vi "系统设置.vi"() -> ()   [LabVIEW 2016]
uses:
  <vilib>/Utility/miscctls.llb/LVPointTypeDef.ctl
  <vilib>/Utility/config.llb/Read Key (U32).vi
  <vilib>/Utility/config.llb/Write Key (I32).vi
  PLC/PLC.lvlib
  <vilib>/ptbypt/NI_PtbyPt.lvlib
  <vilib>/Utility/config.llb/NI_LVConfig.lvlib
panel:
  in  "采水模式":enum16{"使用采水泵", "不使用采水泵"}(ring)
  in  "运行模式":enum16{"维护模式", "常规模式", "应急模式", "质控模式"}(ring)
  in  "运行间隔":i16=4 min=1 max=24
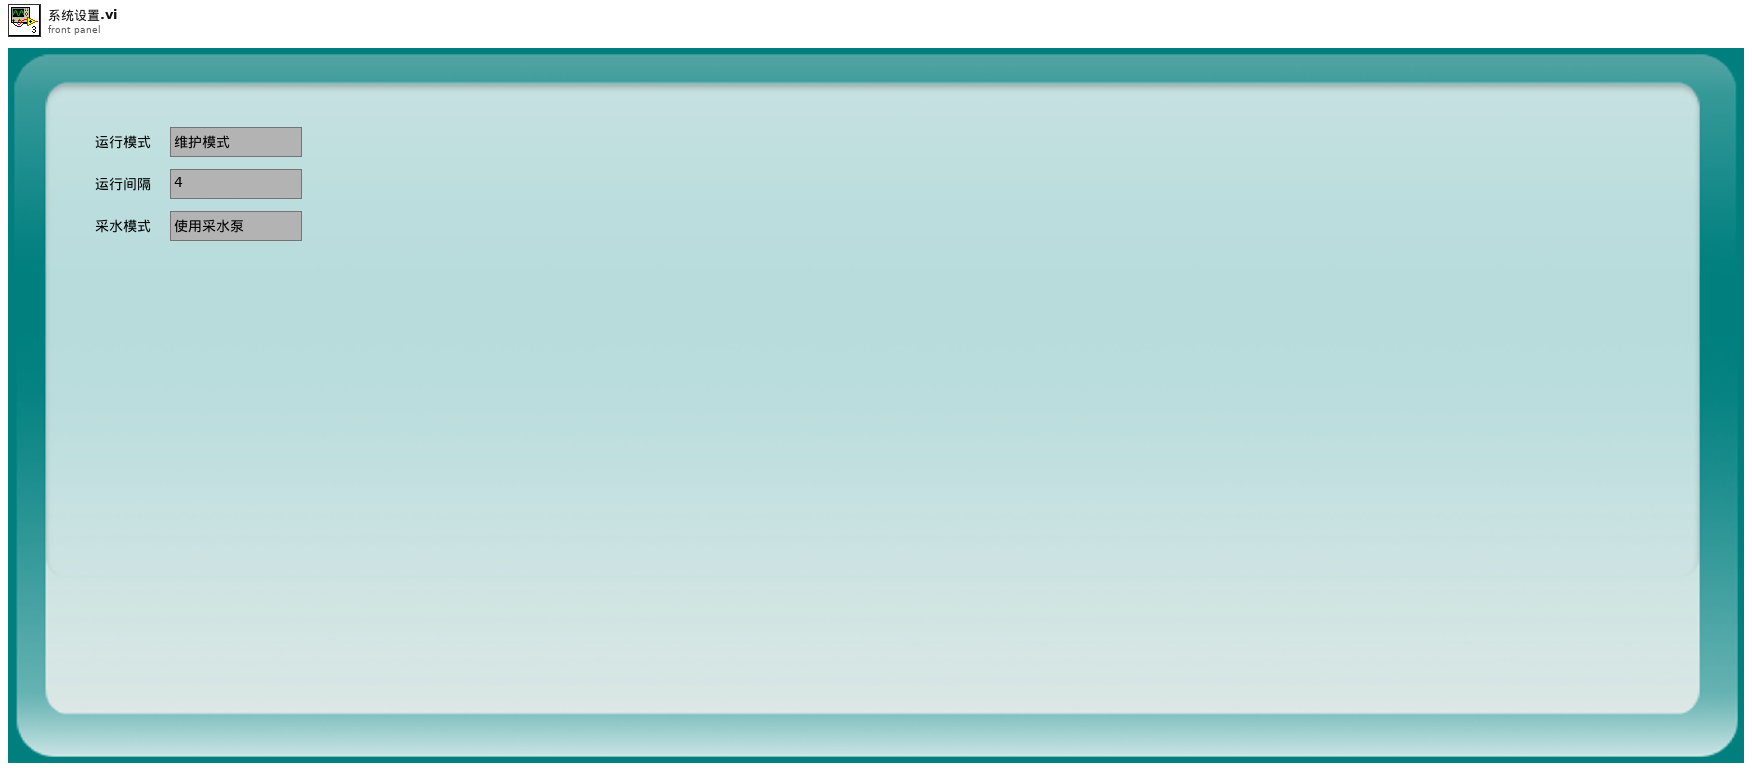
[diagram p1: front panel]
types:
  T1 = typedef "LVPointTypeDef.ctl" = cluster{"Horizontal":i16, "Vertical":i16}
  T2 = typedef "NI_LVConfig.lvlib/Config Data RefNum.ctl" = refnum<k1>
  T3 = enum16{"水样测量", "标样核查", "零点核查", "加标回收", "平行样", "校零", "校标"}
  T4 = cluster{"是否启用仪器":bool, "CODMn":cluster{"启动测量模式":cluster{"测量模式":enum16{"水样测量", "标样核查", "零点核查", "加标回收", "平行样", "校零", "校标"}}, "确定按钮":bool}, "CODCr":cluster{"启动测量模式":cluster{"测量模式":enum16{"水样测量", "标样核查", "零点核查", "加标回收", "平行样", "校零", "校标"}}}, "采水模式":enum16{"使用采水泵", "不使用采水泵"}}
  T5 = typedef "LVDateTimeRec.ctl" = cluster{"秒数的小数部分":dbl, "秒":i32, "分":i32, "时":i32, "日":i32, "月":i32, "年":i32, "天数（周）":i32, "天数（年）":i32, "DST":i32}
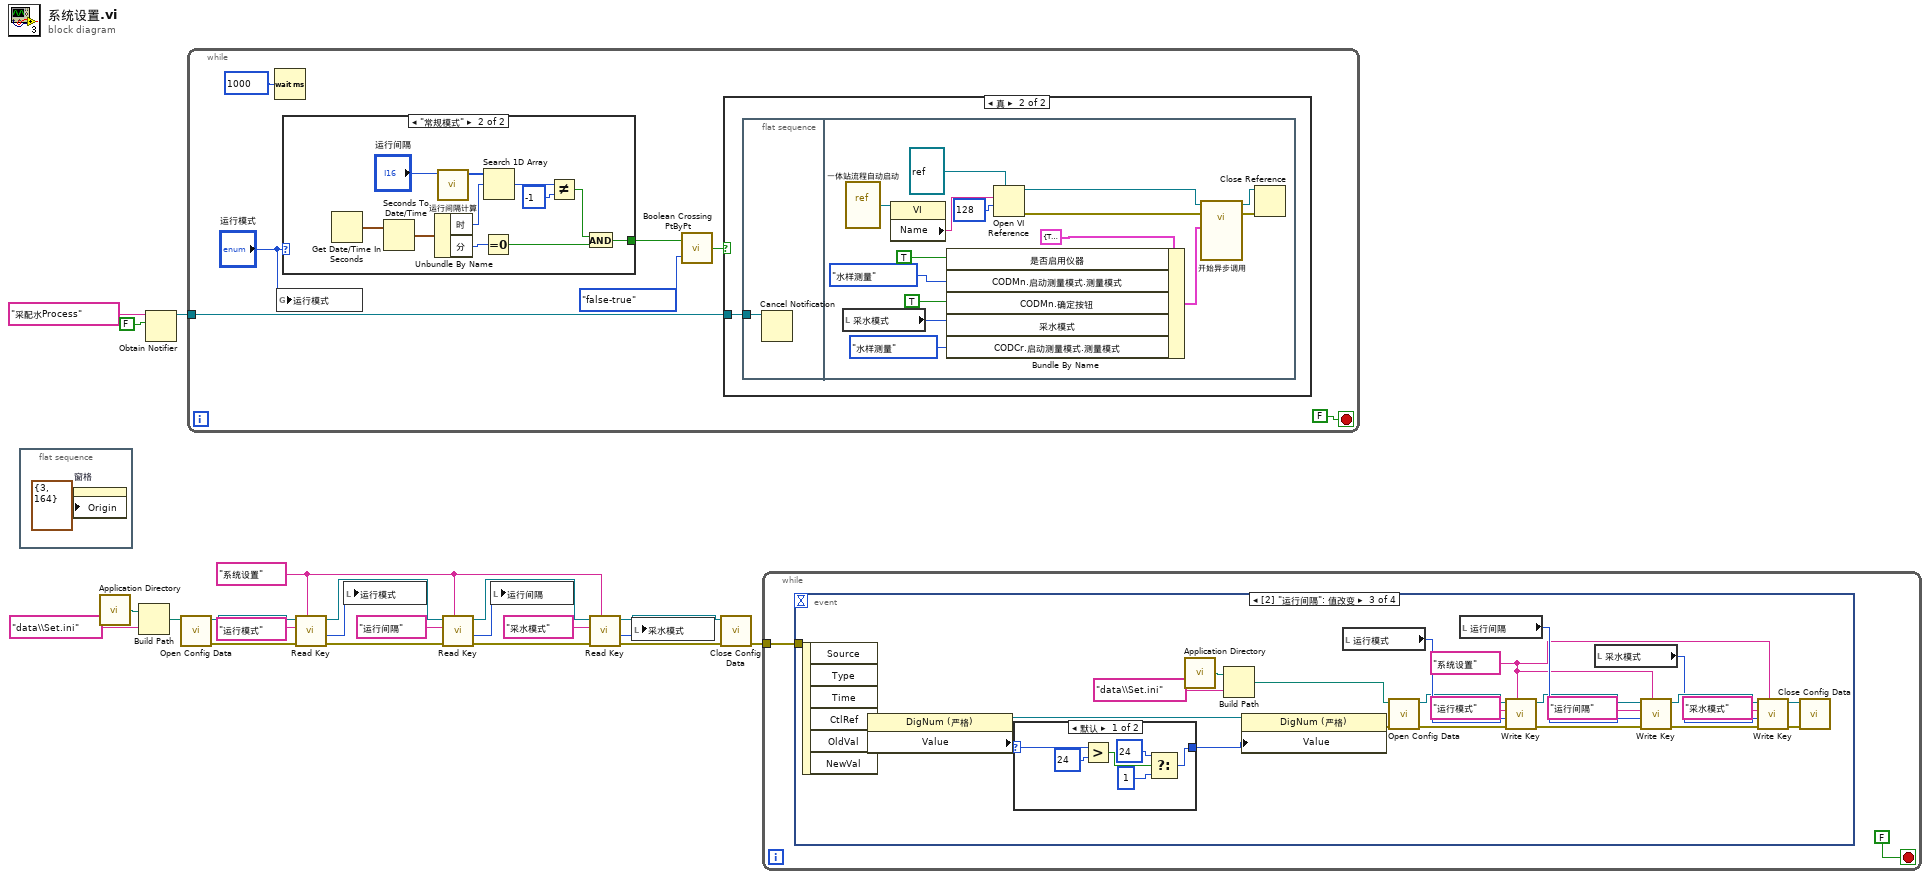
[diagram p0: block diagram]
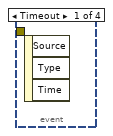
[diagram p4: hidden frame]
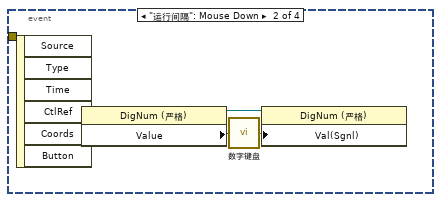
[diagram p5: hidden frame]
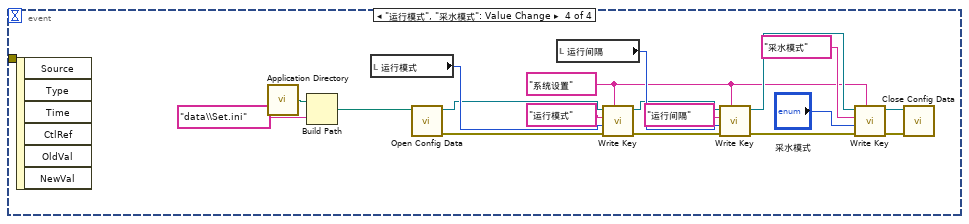
[diagram p7: hidden frame]
diagram:
  w3 = "系统设置" ("section")
  n1 = flat-sequence {
    frame #0 {
      n2 = property on="窗格" class="Pane"("Origin"=T1 {"Horizontal"=3, "Vertical"=164} ("原点")) -> ()  [unwired: 2 in, 2 out]
    }
  }
  n3 = call <vilib>:"Application Directory.vi"() -> ("Application Directory"=w17:path)
  n4 = Build Path(base path=w17, name or relative path="data\\Set.ini" ("名称或相对路径")) -> (appended path=w15:path)
  n5 = Obtain Notifier(name (unnamed)="采配水Process" ("名称（未命名）"), notification data type=FALSE) -> (notifier out=w20:refnum<notifier>)  [unwired: 2 in, 2 out]
  n6 = call <vilib>:"Open Config Data.vi"("configuration file path"=w15) -> ("error out"=w18:errorcluster, "refnum"=w19:T2)  [unwired: 8 in, 1 out]
  n7 = while {
    tunnel: w20 -> [w28]
    stop <- FALSE stop-if-true
    n8 = Wait (ms)(milliseconds to wait=u32 1000 ("等待时间（毫秒）")) -> ()  [unwired: 1 out]
    n9 = global write "系统变量.vi" "运行模式"("运行模式") -> ()
    n10 = case shown="\"常规模式\"" "运行模式" {
      tunnel: [_ w48] -> w27
      frame "维护模式", Default {
      }
      frame "常规模式" {
        n11 = Get Date/Time In Seconds() -> (seconds since 1Jan1904=w57:timestamp)
        n12 = Seconds To Date/Time(time stamp (now)=w57) -> (date time rec=w56:T5)  [unwired: 1 in]
        n13 = Unbundle By Name(w56) -> ("时"=w53:i32, "分"=w55:i32)
        n14 = call "运行间隔计算.vi"("运行周期"="运行间隔") -> ("数组"=w54:i32[])  [unwired: 10 in]
        n15 = Equal To 0?(x=w55) -> (x = 0?=w49:bool)
        n16 = Search 1D Array(1D array=w54, element=w53) -> (index of element=w52:i32)  [unwired: 1 in]
        n17 = Not Equal?(x=w52, y=-1) -> (x != y?=w50:bool)
        n18 = And(x=w50, y=w49) -> (x .and. y?=w48:bool)
      }
    }
    n19 = call <vilib>:"Boolean Crossing PtByPt.vi"("direction"=enum16{"either", "false-true", "true-false"}."false-true", "input"=w27) -> ("crossing"=w25:bool)  [unwired: 1 in]
    n20 = case shown="真" w25 {
      tunnel: w28 -> [_ w31]
      frame False {
      }
      frame True {
        n21 = flat-sequence {
          tunnel: w31 -> [w32]
          frame #0 {
            n22 = Cancel Notification(0:w32) -> ()  [unwired: 1 in, 3 out]
          }
          frame #1 {
            n23 = local read "采水模式"() -> (w36:enum16{"使用采水泵", "不使用采水泵"})
            n24 = vi-ref "一体站流程自动启动.vi"() -> (w47:refnum<vi>)
            n25 = property class="VI"(reference=w47) -> ("Name"=w46:string)  [unwired: 1 in, 2 out]
            n26 = Bundle By Name(cluster=T4 {"是否启用仪器"=TRUE, "CODMn"={"启动测量模式"={"测量模式"=enum."水样测量"}, "确定按钮"=TRUE}, "CODCr"={"启动测量模式"={"测量模式"=enum."水样测量"}}, "采水模式"=enum."使用采水泵"} ("参数"), "是否启用仪器"=TRUE, "CODMn.启动测量模式.测量模式"=T3."水样测量", "CODMn.确定按钮"=TRUE, "采水模式"=w36, "CODCr.启动测量模式.测量模式"=T3."水样测量") -> (w33:T4)
            n27 = Open VI Reference(type specifier VI Refnum (for type only)=refnum<vi> refnum, vi path=w46, options=128 ("选项")) -> (vi reference=w44:refnum<vi>, error out=w41:errorcluster)  [unwired: 3 in]
            n28 = call-by-ref "开始异步调用"(reference=w44, error in=w41, "参数"=w33) -> (reference out=w42:refnum<vi>, error out=w40:errorcluster)  [unwired: 11 in]
            n29 = Close Reference(reference=w42, error in (no error)=w40) -> ()  [unwired: 1 out]
          }
        }
      }
    }
  }
  n30 = call-poly <vilib>:"Read Key.vi"("section"=w3, "error in (no error)"=w18, "key"="运行模式" ("section"), "refnum"=w19) -> ("error out"=w12:errorcluster, "value"=w14:u32, "refnum out"=w13:T2)  [unwired: 4 in, 1 out]
  n31 = local write "运行模式"(w14) -> ()
  n32 = call-poly <vilib>:"Read Key.vi"("section"=w3, "error in (no error)"=w12, "key"="运行间隔" ("section"), "refnum"=w13) -> ("error out"=w6:errorcluster, "value"=w9:u32, "refnum out"=w7:T2)  [unwired: 4 in, 1 out]
  n33 = local write "运行间隔"(w9) -> ()
  n34 = call-poly <vilib>:"Read Key.vi"("section"=w3, "error in (no error)"=w6, "key"="采水模式", "refnum"=w7) -> ("error out"=w4:errorcluster, "value"=w1:u32, "refnum out"=w5:T2)  [unwired: 4 in, 1 out]
  n35 = local write "采水模式"(w1) -> ()
  n36 = call <vilib>:"Close Config Data.vi"("error in (no error)"=w4, "refnum"=w5) -> ("error out"=w8:errorcluster)  [unwired: 8 in, 1 out]
  n37 = while {
    tunnel: w8 -> [w59]
    stop <- FALSE stop-if-true
    n38 = event shown="[2] \"运行间隔\": 值改变" {
      selector: _ -> [_ _ _ _]
      dyn-events: _ -> [_ _ _ _]
      timeout: _ -> [_ _ _ _]
      tunnel: w59 -> [_ _ _ _]
      event Timeout {
        n39 = event-data() -> ()  [unwired: 1 in, 3 out]
      }
      event "运行间隔": Mouse Down {
        n40 = event-data() -> ("CtlRef"=w61:refnum<vi>)  [unwired: 1 in, 5 out]
        n41 = property class="DigNum (严格)"(reference=w61) -> (reference out=w63:refnum<vi>, "Value"=w62:i16)  [unwired: 1 in, 1 out]
        n42 = call "数字键盘.vi"("OldNumber"=w62) -> ("NewNumber"=w64:sgl)
        n43 = property class="DigNum (严格)"(reference=w63, "Val(Sgnl)"=w64) -> ()  [unwired: 1 in, 2 out]
      }
      event "运行间隔": Value Change {
        w65 = "系统设置" ("section")
        n44 = event-data() -> ("CtlRef"=w87:refnum<vi>)  [unwired: 1 in, 5 out]
        n45 = property class="DigNum (严格)"(reference=w87) -> (reference out=w85:refnum<vi>, "Value"=w86:i16)  [unwired: 1 in, 1 out]
        n46 = case shown="默认" w86 {
          selector: w86 -> [w90 w94]
          tunnel: [w89 w94] -> w84
          frame Default {
            n47 = Greater?(x=w90, y=i16 24) -> (0:w92:bool)
            n48 = Select(t=i16 24 ("y"), s=w92, f=i16 1) -> (s? t:f=w89:i16)
          }
          frame 1..24 {
          }
        }
        n49 = call <vilib>:"Application Directory.vi"() -> ("Application Directory"=w79:path)
        n50 = Build Path(base path=w79, name or relative path="data\\Set.ini" ("名称或相对路径")) -> (appended path=w77:path)
        n51 = property class="DigNum (严格)"(reference=w85, "Value"=w84) -> (error out=w72:errorcluster)  [unwired: 1 in, 1 out]
        n52 = local read "运行模式"() -> (w82:enum16{"维护模式", "常规模式", "应急模式", "质控模式"})
        n53 = call <vilib>:"Open Config Data.vi"("error in (no error)"=w72, "configuration file path"=w77) -> ("error out"=w80:errorcluster, "refnum"=w81:T2)  [unwired: 7 in, 1 out]
        n54 = local read "运行间隔"() -> (w83:i16)
        n55 = call-poly <vilib>:"Write Key.vi"("section"=w65, "error in (no error)"=w80, "value"=w82, "key"="运行模式" ("section"), "refnum"=w81) -> ("error out"=w75:errorcluster, "refnum out"=w76:T2)  [unwired: 4 in, 1 out]
        n56 = local read "采水模式"() -> (w66:enum16{"使用采水泵", "不使用采水泵"})
        n57 = call-poly <vilib>:"Write Key.vi"("section"=w65, "error in (no error)"=w75, "value"=w83, "key"="运行间隔" ("section"), "refnum"=w76) -> ("error out"=w68:errorcluster, "refnum out"=w70:T2)  [unwired: 4 in, 1 out]
        n58 = call-poly <vilib>:"Write Key.vi"("section"=w65, "error in (no error)"=w68, "value"=w66, "key"="采水模式", "refnum"=w70) -> ("error out"=w67:errorcluster, "refnum out"=w69:T2)  [unwired: 4 in, 1 out]
        n59 = call <vilib>:"Close Config Data.vi"("error in (no error)"=w67, "refnum"=w69) -> ()  [unwired: 8 in, 2 out]
      }
      event "运行模式", "采水模式": Value Change {
        w95 = "系统设置" ("section")
        n60 = event-data() -> ()  [unwired: 1 in, 6 out]
        n61 = call <vilib>:"Application Directory.vi"() -> ("Application Directory"=w108:path)
        n62 = Build Path(base path=w108, name or relative path="data\\Set.ini" ("名称或相对路径")) -> (appended path=w106:path)
        n63 = local read "运行模式"() -> (w111:enum16{"维护模式", "常规模式", "应急模式", "质控模式"})
        n64 = call <vilib>:"Open Config Data.vi"("configuration file path"=w106) -> ("error out"=w109:errorcluster, "refnum"=w110:T2)  [unwired: 8 in, 1 out]
        n65 = local read "运行间隔"() -> (w112:i16)
        n66 = call-poly <vilib>:"Write Key.vi"("section"=w95, "error in (no error)"=w109, "value"=w111, "key"="运行模式" ("section"), "refnum"=w110) -> ("error out"=w104:errorcluster, "refnum out"=w105:T2)  [unwired: 4 in, 1 out]
        n67 = call-poly <vilib>:"Write Key.vi"("section"=w95, "error in (no error)"=w104, "value"=w112, "key"="运行间隔" ("section"), "refnum"=w105) -> ("error out"=w97:errorcluster, "refnum out"=w99:T2)  [unwired: 4 in, 1 out]
        n68 = call-poly <vilib>:"Write Key.vi"("section"=w95, "error in (no error)"=w97, "value"="采水模式", "key"="采水模式", "refnum"=w99) -> ("error out"=w96:errorcluster, "refnum out"=w98:T2)  [unwired: 4 in, 1 out]
        n69 = call <vilib>:"Close Config Data.vi"("error in (no error)"=w96, "refnum"=w98) -> ()  [unwired: 8 in, 2 out]
      }
    }
  }
